vi "Global.vi"() -> ()   [LabVIEW 2019, in "GaitDAQ UI.lvlib"]
uses:
  GaitDAQ UI.lvlib
  Status.ctl
  <vilib>/userdefined/High Color/IMAQdx.ctl
  <vilib>/vision/Avi.llb/IMAQ AVI2 Refnum.ctl
panel:
  in  "COM Port":refnum<visa-resource-name>
  in  "Foot File Refnum":refnum<file>
  in  "Camera File Refnum":T1
  in  "Data Folder":path
  in  "Camera Session":T2
  in  "Status":T3=-1 items=["Wait"=-1, "Run"=10, "Play"=33]
  in  "Log？":bool
  in  "Camera Open？":bool
  in  "COM Open？":bool
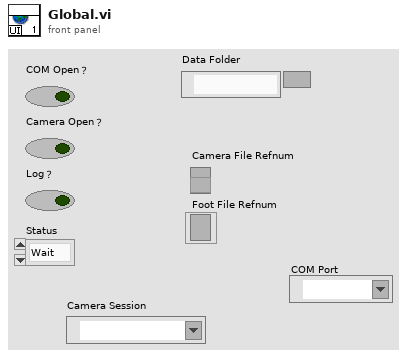
[diagram p1: front panel]
types:
  T1 = typedef "IMAQ AVI2 Refnum.ctl" = refnum<k20>
  T2 = typedef "IMAQdx.ctl" = refnum<k21>
  T3 = typedef "GaitDAQ UI.lvlib/Status.ctl" = i32
diagram:
